vi "Encoders.vi"(1 "Number of Encoders":i32=1 min=1 max=5, 2 "Reset":bool, 3 "Mode":enum8{"Start", "Run", "Finish"}(ring)) -> (0 "Encoder":T1(array[cluster]))   [LabVIEW 2014]
uses:
  <vilib>/Rock Robotics/WPI/Counter/WPI_CounterDigitalInputToDigitalSource.vi
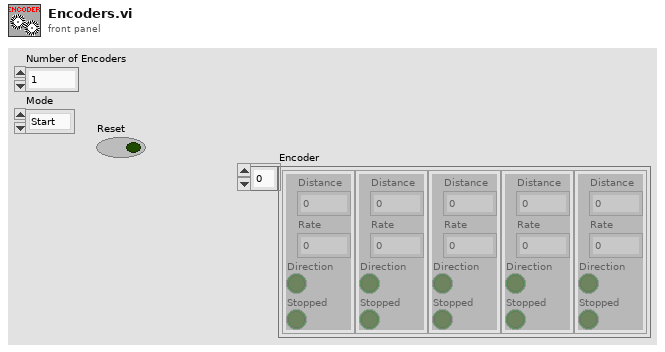
[diagram p1: front panel]
types:
  T1 = cluster{"Distance":dbl, "Rate":dbl, "Direction":bool, "Stopped":bool}[]
  T2 = cluster{"Distance":dbl, "Rate":dbl, "Direction":bool, "Stopped":bool}
  T3 = typedef "WPI_EncoderDevRef.ctl" = cluster{"DevStatus":errorcluster, "EncoderIndex":T4, "CounterIndex":T5, "DistancePerCount":dbl, "Decoding Type":T6}
  T4 = typedef "FPGA_EncoderIdx.ctl" = enum8{"Enc 0", "Enc 1", "Enc 2", "Enc 3", "Enc 4", "Enc 5", "Enc 6", "Enc 7", "Invalid"}
  T5 = typedef "FPGA_CounterCtrSystemIndex.ctl" = enum8{"Ctr 0", "Ctr 1", "Ctr 2", "Ctr 3", "Ctr 4", "Ctr 5", "Ctr 6", "Ctr 7", "Invalid"}
  T6 = typedef "WPI_EncoderType.ctl" = enum16{"1x", "2x", "4x"}
  T7 = typedef "WPI_DigitalInputDevRef.ctl" = cluster{"DevStatus":errorcluster, "DIO Channel":T8, "Controller":T9}
  T8 = typedef "FPGA_DIOChannel.ctl" = enum8{"DIO 0", "DIO 1", "DIO 2", "DIO 3", "DIO 4", "DIO 5", "DIO 6", "DIO 7", "DIO 8", "DIO 9", "DIO MXP 0", "DIO MXP 1", "DIO MXP 2", "DIO MXP 3", "DIO MXP 4", "DIO MXP 5", "DIO MXP 6", "DIO MXP 7", "DIO MXP 8", "DIO MXP 9", "DIO MXP 10", "DIO MXP 11", "DIO MXP 12", "DIO MXP 13", "DIO MXP 14", "DIO MXP 15", "Invalid"}
  T9 = typedef "FPGA_TypedefDigitalModule.ctl" = enum16{"Controller 1"}
  T10 = typedef "FPGA_CounterEncoderSourceConvertionLVSourceType.ctl" = cluster{"DevStatus":errorcluster, "AnalogTriggerMode?":bool, "DigitalMode":cluster{"Controller":T9, "DIO Channel":T11}, "AnalogTriggerMode":cluster{"AnalogTriggerIndex":T12, "OutputType":T13}}
  T11 = typedef "FPGA_DIODigitalSourceChannel.ctl" = enum8{"DIO 0", "DIO 1", "DIO 2", "DIO 3", "DIO 4", "DIO 5", "DIO 6", "DIO 7", "DIO 8", "DIO 9", "DIO MXP 0", "DIO MXP 1", "DIO MXP 2", "DIO MXP 3", "DIO MXP 4", "DIO MXP 5", "DIO MXP 6", "DIO MXP 7", "DIO MXP 8", "DIO MXP 9", "DIO MXP 10", "DIO MXP 11", "DIO MXP 12", "DIO MXP 13", "DIO MXP 14", "DIO MXP 15", "Disabled"}
  T12 = typedef "FPGA_AnalogTriggerIndex.ctl" = enum8{"Trig 0", "Trig 1", "Trig 2", "Trig 3", "Trig 4", "Trig 5", "Trig 6", "Trig 7", "Invalid"}
  T13 = typedef "FPGA_AnalogTriggerOutType.ctl" = enum16{"InWindow", "TriggerState", "Rising", "Falling"}
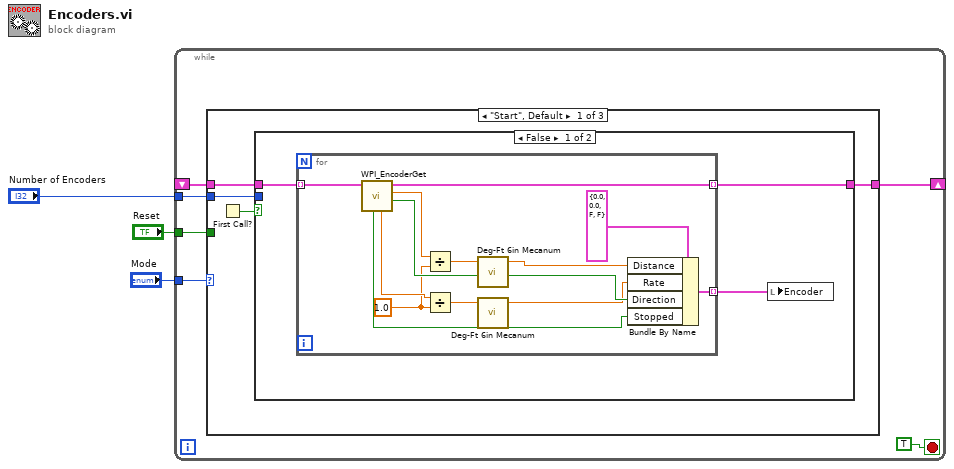
[diagram p0: block diagram]
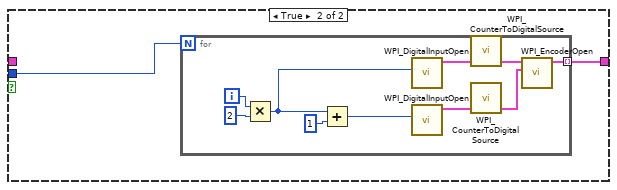
[diagram p2: hidden frame]
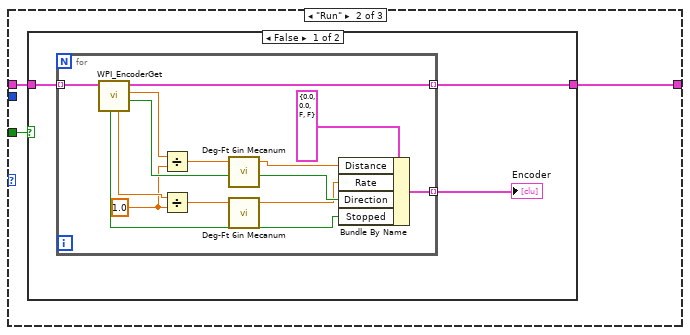
[diagram p3: hidden frame]
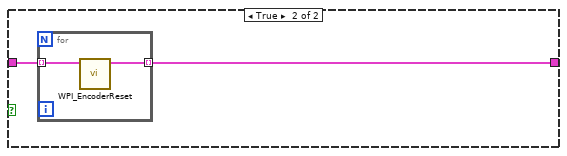
[diagram p4: hidden frame]
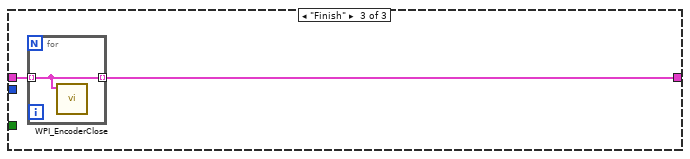
[diagram p5: hidden frame]
diagram:
  n1 = while {
    tunnel: "Number of Encoders" -> [w9]
    tunnel: "Mode" -> [w8]
    shift-right: [w7] -> _
    shift-left: _ -> [w6]
    tunnel: "Reset" -> [w4]
    stop <- TRUE stop-if-true
    n2 = case shown="\"Start\", Default" w8 {
      tunnel: w9 -> [w13 _ _]
      tunnel: [w12 w43 w65] -> w7
      tunnel: w6 -> [w10 w44 w66]
      tunnel: w4 -> [_ w42 _]
      frame "Start", Default {
        n3 = First Call?() -> (First Call?: T/F=w11:bool)
        n4 = case shown="False" w11 {
          tunnel: w13 -> [_ w31]
          tunnel: [w15 w30] -> w12
          tunnel: w10 -> [w16 _]
          frame False {
            n5 = for {
              tunnel: w16 -> [w29] mode=indexing
              tunnel: [w28] -> w15 mode=indexing
              tunnel: [w24] -> w14 mode=indexing
              w21 = 1.0 ("y")
              n6 = call <vilib>:"WPI_EncoderGet.vi"("EncoderDevRef"=w29) -> ("Direction"=w26:bool, "Distance"=w23:dbl, "EncoderDevRef"=w28:T3, "Rate"=w22:dbl, "Stopped"=w25:bool)  [unwired: 5 in, 1 out]
              n7 = Divide(x=w23, y=w21) -> (x/y=w19:dbl)
              n8 = Divide(x=w22, y=w21) -> (x/y=w20:dbl)
              n9 = call "Deg-Ft 6in Mecanum.vi"("Input"=w19) -> ("Output"=w18:dbl)  [unwired: 4 in]
              n10 = call "Deg-Ft 6in Mecanum.vi"("Input"=w20) -> ("Output"=w17:dbl)  [unwired: 4 in]
              n11 = Bundle By Name(cluster=T2 {"Distance"=0.0, "Rate"=0.0, "Direction"=FALSE, "Stopped"=FALSE} ("Encoder"), "Distance"=w18, "Rate"=w17, "Direction"=w26, "Stopped"=w25) -> (w24:T2)
            }
            n12 = local write "Encoder"(w14) -> ()
          }
          frame True {
            n13 = for {
              N: w31 -> [_]
              tunnel: [w32] -> w30 mode=indexing
              i -> [w37]
              n14 = Multiply(x=w37, y=2) -> (x*y=w34:i32)
              n15 = Add(x=w34, y=1) -> (x+y=w35:i32)
              n16 = call <vilib>:"WPI_DigitalInputOpen.vi"("DIO Channel"=w34) -> ("DigitalInputDevRef"=w39:T7)  [unwired: 2 in, 8 out]
              n17 = call <vilib>:"WPI_DigitalInputOpen.vi"("DIO Channel"=w35) -> ("DigitalInputDevRef"=w40:T7)  [unwired: 2 in, 8 out]
              n18 = call-poly <vilib>:"WPI_CounterToDigitalSource.vi"("DigitalInputDevRef"=w39) -> ("Digital Source"=w38:T10)  [unwired: 6 out]
              n19 = call-poly <vilib>:"WPI_CounterToDigitalSource.vi"("DigitalInputDevRef"=w40) -> ("Digital Source"=w41:T10)  [unwired: 6 out]
              n20 = call <vilib>:"WPI_EncoderOpen.vi"("BSource"=w41, "ASource"=w38) -> ("EncoderDevRef"=w32:T3)  [unwired: 6 in, 3 out]
            }
          }
        }
      }
      frame "Run" {
        n21 = case shown="False" w42 {
          tunnel: w44 -> [w47 w62]
          tunnel: [w46 w61] -> w43
          frame False {
            n22 = for {
              tunnel: w47 -> [w60] mode=indexing
              tunnel: [w59] -> w46 mode=indexing
              tunnel: [w55] -> w45 mode=indexing
              w52 = 1.0 ("y")
              n23 = call <vilib>:"WPI_EncoderGet.vi"("EncoderDevRef"=w60) -> ("Direction"=w57:bool, "Distance"=w54:dbl, "EncoderDevRef"=w59:T3, "Rate"=w53:dbl, "Stopped"=w56:bool)  [unwired: 5 in, 1 out]
              n24 = Divide(x=w54, y=w52) -> (x/y=w50:dbl)
              n25 = Divide(x=w53, y=w52) -> (x/y=w51:dbl)
              n26 = call "Deg-Ft 6in Mecanum.vi"("Input"=w50) -> ("Output"=w49:dbl)  [unwired: 4 in]
              n27 = call "Deg-Ft 6in Mecanum.vi"("Input"=w51) -> ("Output"=w48:dbl)  [unwired: 4 in]
              n28 = Bundle By Name(cluster=T2 {"Distance"=0.0, "Rate"=0.0, "Direction"=FALSE, "Stopped"=FALSE} ("Encoder"), "Distance"=w49, "Rate"=w48, "Direction"=w57, "Stopped"=w56) -> (w55:T2)
            }
            "Encoder" <- w45
          }
          frame True {
            n29 = for {
              tunnel: [w63] -> w61 mode=indexing
              tunnel: w62 -> [w64] mode=indexing
              n30 = call <vilib>:"WPI_EncoderReset.vi"("EncoderDevRef"=w64) -> ("EncoderDevRef"=w63:T3)  [unwired: 9 in, 1 out]
            }
          }
        }
      }
      frame "Finish" {
        n31 = for {
          tunnel: [w67] -> w65 mode=indexing
          tunnel: w66 -> [w67] mode=indexing
          n32 = call <vilib>:"WPI_EncoderClose.vi"("EncoderDevRef"=w67) -> ()  [unwired: 10 in, 1 out]
        }
      }
    }
  }
